vi "DI Coil UI.vi"(8 "error in (no error)":errorcluster, 11 "Node Ptr":T1 format="%.0x") -> (0 "error out":errorcluster)   [LabVIEW 2021, in "Modbus Master System Explorer.lvlib"]
uses:
  Modbus Master System Explorer.lvlib
  <vilib>/NI VeriStand/Custom Device API/Custom Device Item Ref.ctl
  SubVIs/Modbus Type.ctl
  <vilib>/NI VeriStand/Custom Device API/Custom Device API.lvlib
  Shared/Modbus Master Shared.lvlib
panel:
  in  "Unit ID":u8
  in  "Address":u16
  in  "Valid?":string
  in  "Header":cluster{"Section Name":string}={"Section Name"="Discrete Input Settings"}
  in  "Description":string
  in  "Name":string
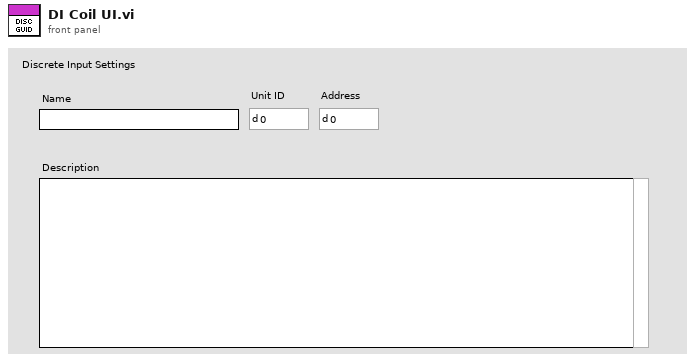
[diagram p1: front panel]
types:
  T1 = typedef "Custom Device API.lvlib/Custom Device Item Ref.ctl" = u64
  T2 = typedef "Modbus Master Shared.lvlib/Modbus Type.ctl" = enum16{"Coil", "Discrete Input", "Holding Register", "Input Register"}
  T3 = typedef "Custom Device API.lvlib/Custom Device Commands.ctl" = enum16{"Default", "Item renamed", "Shutdown", "Dynamic button pressed"}
  T4 = typedef "Custom Device API.lvlib/Custom Device Item Info.ctl" = cluster{"Name":string, "Is Channel":bool, "GUID":string, "Is Waveform":bool}
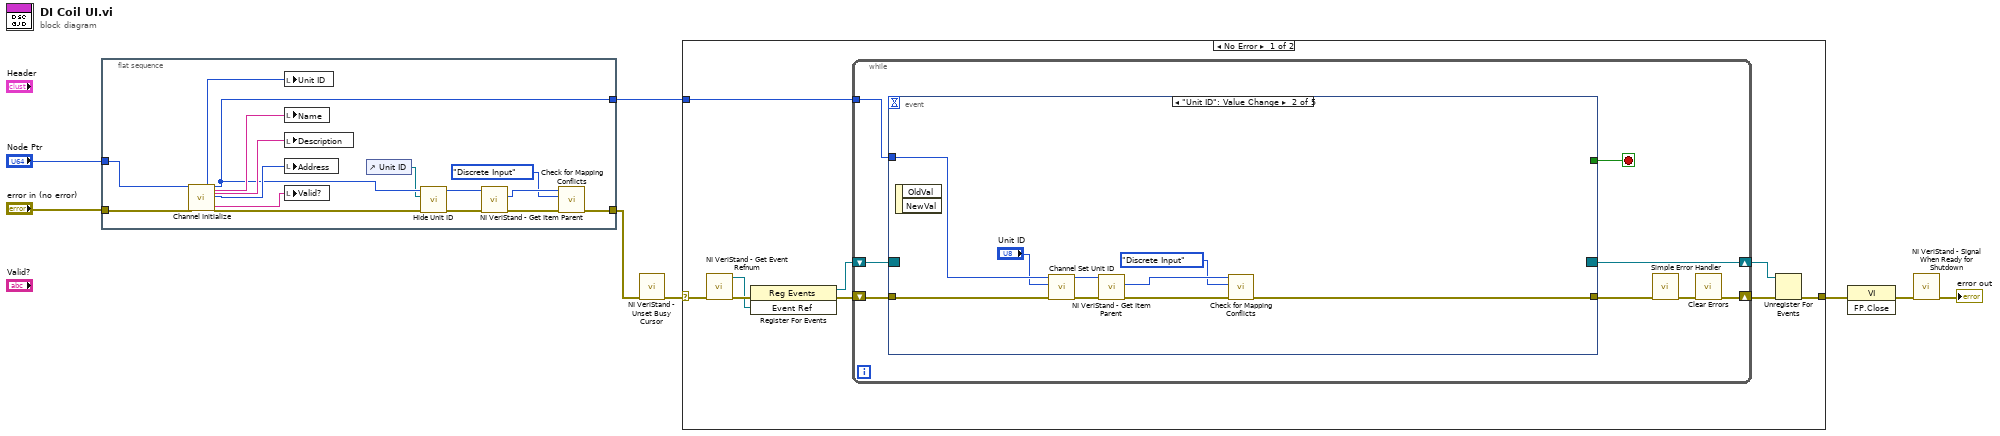
[diagram p0: block diagram]
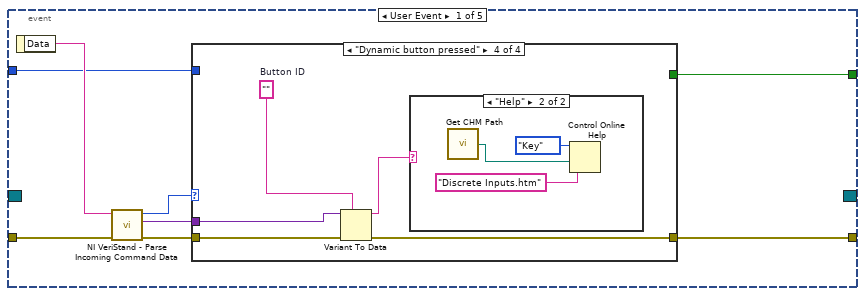
[diagram p2: hidden frame]
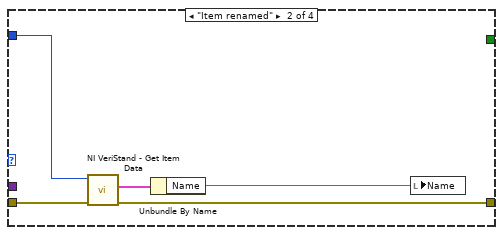
[diagram p4: hidden frame]
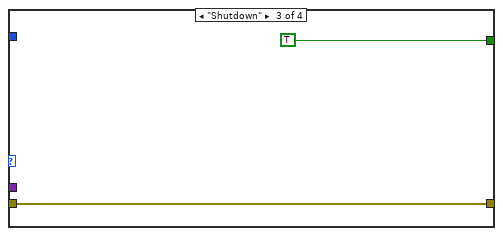
[diagram p5: hidden frame]
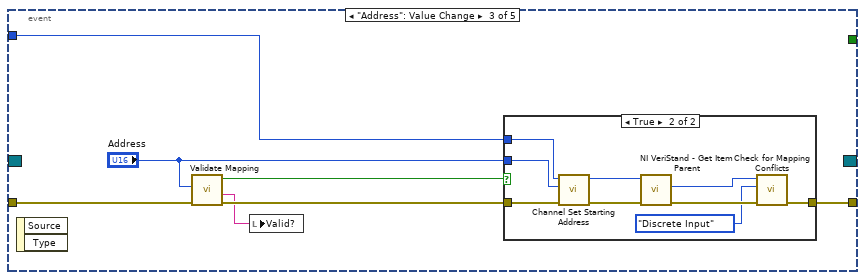
[diagram p7: hidden frame]
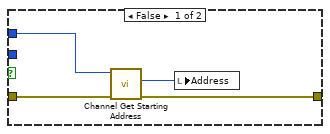
[diagram p8: hidden frame]
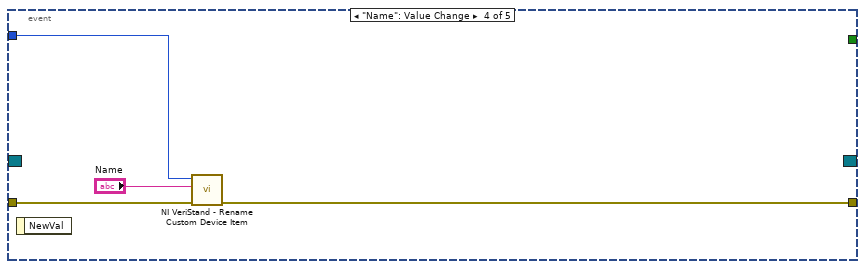
[diagram p9: hidden frame]
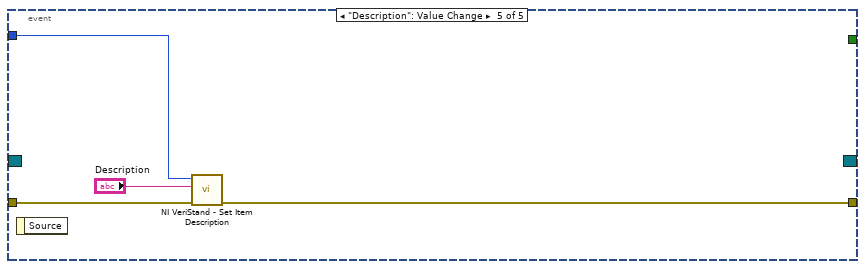
[diagram p10: hidden frame]
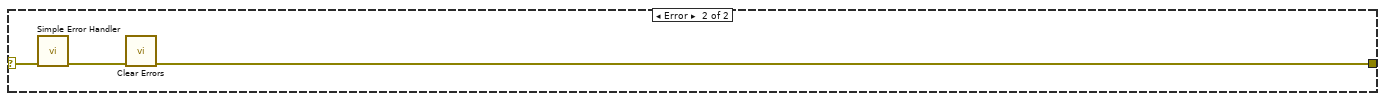
[diagram p11: hidden frame]
diagram:
  n1 = flat-sequence {
    tunnel: "Node Ptr" -> [w21]
    tunnel: [w13] -> w3
    tunnel: "error in (no error)" -> [w20]
    tunnel: [w14] -> w1
    frame #0 {
      n2 = call "Channel Initialize.vi"("Item Ref in"=w21, "error in (no error)"=w20) -> ("Unit ID"=w18:u8, "Channel Ref out"=w13:T1, "Name"=w23:string, "Description"=w22:string, "Starting Address"=w19:u16, "Status Message"=w24:string, "error out"=w11:errorcluster)  [unwired: 13 in, 6 out]
      n3 = local write "Unit ID"(w18) -> ()
      n4 = local write "Name"(w23) -> ()
      n5 = local write "Description"(w22) -> ()
      n6 = local write "Address"(w19) -> ()
      n7 = local write "Valid?"(w24) -> ()
      n8 = control-ref of="Unit ID"() -> (w9:refnum<vi>)
      n9 = call "Hide Unit ID.vi"("error in (no error)"=w11, "Ctrl Ref"=w9, "Item Ref in"=w13) -> ("error out"=w10:errorcluster, "Item Ref out"=w12:T1)  [unwired: 7 in]
      n10 = call <vilib>:"NI VeriStand - Get Item Parent.vi"("error in (no error)"=w10, "Item Ref in"=w12) -> ("error out"=w15:errorcluster, "Parent Ref"=w17:T1)  [unwired: 6 in, 2 out]
      n11 = call "Check for Mapping Conflicts.vi"("error in (no error)"=w15, "Type"=Modbus_Type."Discrete Input", "Coiil Group Ref in in"=w17) -> ("error out"=w14:errorcluster)  [unwired: 5 in, 3 out]
    }
  }
  n12 = call <vilib>:"NI VeriStand - Unset Busy Cursor.vi"("error in (no error)"=w1) -> ("error out"=w5:errorcluster)  [unwired: 10 out]
  n13 = case shown="No Error" w5 {
    selector: w5 -> [w25 w105]
    tunnel: [w30 w103] -> w8
    tunnel: w3 -> [w26 _]
    frame No Error {
      n14 = call <vilib>:"NI VeriStand - Get Event Refnum.vi"("error in (no error)"=w25) -> ("error out"=w33:errorcluster, "Event Ref"=w29:refnum<user-event>)  [unwired: 9 out]
      n15 = register-events(error in=w33, w29) -> (reference out=w27:refnum<event-registration>, error out=w28:errorcluster)  [unwired: 1 in]
      n16 = while {
        tunnel: w26 -> [w37]
        shift-right: [w34] -> w31
        shift-left: w28 -> [w40]
        shift-right: [w41] -> w32
        shift-left: w27 -> [w39]
        stop <- w38 stop-if-true
        n17 = event shown="[1] \"Unit ID\": Value Change" {
          selector: w39 -> [_ _ _ _ _]
          dyn-events: [_ _ _ _ _] -> w41
          timeout: _ -> [_ _ _ _ _]
          tunnel: w40 -> [w49 w72 w78 w98 w101]
          tunnel: [w45 _ _ _ _] -> w38
          tunnel: [w44 w66 w80 w97 w100] -> w36
          tunnel: w37 -> [w43 w74 w81 w96 w102]
          event User Event {
            n18 = event-data() -> ("Data"=w48:string)  [unwired: 1 out]
            n19 = call <vilib>:"NI VeriStand - Parse Incoming Command Data.vi"("error in (no error)"=w49, "Incoming data"=w48) -> ("error out"=w47:errorcluster, "Outgoing data"=w42:variant, "Action"=w46:T3)  [unwired: 7 out]
            n20 = case shown="\"Dynamic button pressed\"" w46 {
              tunnel: w47 -> [w50 w55 w56 w62]
              tunnel: [_ _ TRUE _] -> w45
              tunnel: [w50 w52 w56 w59] -> w44
              tunnel: w43 -> [_ w54 _ _]
              tunnel: w42 -> [_ _ _ w61]
              frame "Default", Default {
              }
              frame "Item renamed" {
                n21 = call <vilib>:"NI VeriStand - Get Item Data.vi"("error in (no error)"=w55, "Item Ref in"=w54) -> ("error out"=w52:errorcluster, "Item Info"=w53:T4)  [unwired: 8 out]
                n22 = Unbundle By Name(w53) -> ("Name"=w51:string)
                n23 = local write "Name"(w51) -> ()
              }
              frame "Shutdown" {
              }
              frame "Dynamic button pressed" {
                w60 = ""  # Button ID
                n24 = Variant To Data(error in=w62, type=w60, Variant=w61) -> (data=w58:string, error out=w59:errorcluster)
                n25 = case shown="\"Help\"" w58 {
                  frame Default {
                  }
                  frame "Help" {
                    n26 = call "Get CHM Path.vi"() -> ("appended path"=w65:path)
                    n27 = Control Online Help(2:w65, 3:"Discrete Inputs.htm" ("String to search for"), 4:enum16{"Contents", "Key", "Close"}."Key" ("Operation")) -> ()  [unwired: 1 in, 1 out]
                  }
                }
              }
            }
          }
          event "Unit ID": Value Change {
            n28 = event-data() -> ()  [unwired: 3 out]
            n29 = call "Channel Set Unit ID.vi"("error in (no error)"=w72, "Value"="Unit ID", "Item Ref in"=w74) -> ("error out"=w67:errorcluster, "Item Ref out"=w68:T1)  [unwired: 7 in]
            n30 = call <vilib>:"NI VeriStand - Get Item Parent.vi"("error in (no error)"=w67, "Item Ref in"=w68) -> ("error out"=w70:errorcluster, "Parent Ref"=w71:T1)  [unwired: 6 in, 2 out]
            n31 = call "Check for Mapping Conflicts.vi"("error in (no error)"=w70, "Type"=Modbus_Type."Discrete Input", "Coiil Group Ref in in"=w71) -> ("error out"=w66:errorcluster)  [unwired: 5 in, 3 out]
          }
          event "Address": Value Change {
            n32 = event-data() -> ()  [unwired: 3 out]
            n33 = call "Validate Mapping.vi"("error in (no error)"=w78, "Mapping"="Address") -> ("error out"=w77:errorcluster, "Status Message"=w76:string, "Valid?"=w79:bool)  [unwired: 7 in]
            n34 = local write "Valid?"(w76) -> ()
            n35 = case shown="True" w79 {
              tunnel: w81 -> [w83 w94]
              tunnel: w77 -> [w85 w93]
              tunnel: [w84 w89] -> w80
              tunnel: "Address" -> [_ w87]
              frame False {
                n36 = call "Channel Get Starting Address.vi"("error in (no error)"=w85, "Item Ref in"=w83) -> ("error out"=w84:errorcluster, "Value"=w82:u16)  [unwired: 7 in, 1 out]
                n37 = local write "Address"(w82) -> ()
              }
              frame True {
                n38 = call "Channel Set Starting Address.vi"("error in (no error)"=w93, "Value"=w87, "Item Ref in"=w94) -> ("error out"=w92:errorcluster, "Item Ref out"=w88:T1)  [unwired: 7 in]
                n39 = call <vilib>:"NI VeriStand - Get Item Parent.vi"("error in (no error)"=w92, "Item Ref in"=w88) -> ("error out"=w90:errorcluster, "Parent Ref"=w91:T1)  [unwired: 6 in, 2 out]
                n40 = call "Check for Mapping Conflicts.vi"("error in (no error)"=w90, "Type"=Modbus_Type."Discrete Input", "Coiil Group Ref in in"=w91) -> ("error out"=w89:errorcluster)  [unwired: 5 in, 3 out]
              }
            }
          }
          event "Name": Value Change {
            n41 = event-data() -> ()  [unwired: 2 out]
            n42 = call <vilib>:"NI VeriStand - Rename Custom Device Item.vi"("error in (no error)"=w98, "New Name"="Name", "Item Ref in"=w96) -> ("error out"=w97:errorcluster)  [unwired: 1 in, 7 out]
          }
          event "Description": Value Change {
            n43 = event-data() -> ()  [unwired: 2 out]
            n44 = call <vilib>:"NI VeriStand - Set Item Description.vi"("error in (no error)"=w101, "Description"="Description", "Item Ref in"=w102) -> ("error out"=w100:errorcluster)  [unwired: 8 out]
          }
        }
        n45 = call <vilib>:"Simple Error Handler.vi"("error in (no error)"=w36) -> ("error out"=w35:errorcluster)  [unwired: 1 in, 7 out]
        n46 = call <vilib>:"Clear Errors.vi"("error in (no error)"=w35) -> ("error out"=w34:errorcluster)  [unwired: 1 in, 5 out]
      }
      n47 = Unregister For Events(event registration refnum=w32, error in=w31) -> (error out=w30:errorcluster)
    }
    frame Error {
      n48 = call <vilib>:"Simple Error Handler.vi"("error in (no error)"=w105) -> ("error out"=w104:errorcluster)  [unwired: 1 in, 7 out]
      n49 = call <vilib>:"Clear Errors.vi"("error in (no error)"=w104) -> ("error out"=w103:errorcluster)  [unwired: 1 in, 5 out]
    }
  }
  n50 = invoke class="VI" method="FP.Close"(error in=w8) -> (error out=w7:errorcluster)  [unwired: 2 in, 2 out]
  n51 = call <vilib>:"NI VeriStand - Signal When Ready for Shutdown.vi"("error in (no error)"=w7) -> ("error out"=→"error out":errorcluster)  [unwired: 10 out]
